vi "Read Dashboard Variables.vi"() -> ()   [LabVIEW 2020]
uses:
  <vilib>/Rock Robotics/Network Tables/NT Read Number.vi
  Framework/Robot Global Data.vi
panel:
  out "Transfer Release Duration":dbl
  out "Transfer Up Duration":dbl
  out "Intake Duration":dbl
  out "Shooter Duration":dbl
  out "Transfer Release Setpoint":dbl
  out "Transfer Up Setpoint":dbl
  out "Intake Setpoint":dbl
  out "Shooter Setpoint":dbl
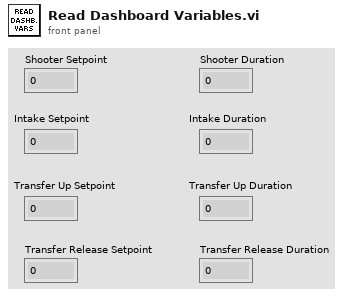
[diagram p1: front panel]
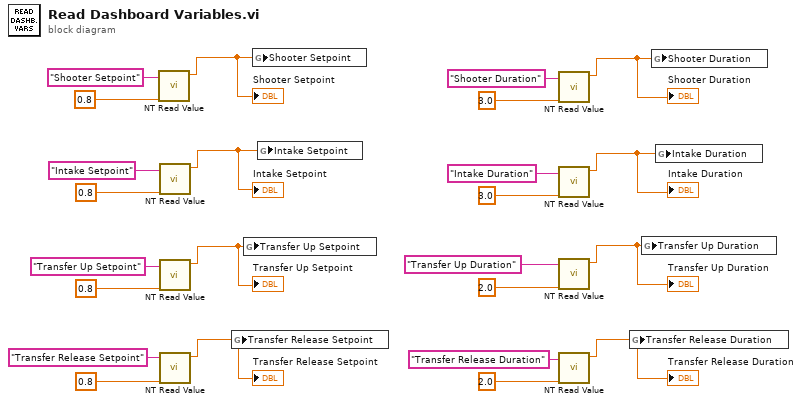
[diagram p0: block diagram]
diagram:
  n1 = call-poly <vilib>:"NT Read Value.vi"("Default Value"=0.8, "Name"="Shooter Setpoint") -> ("Numeric"=w22:dbl)  [unwired: 8 in, 1 out]
  "Shooter Setpoint" <- w22
  n2 = call-poly <vilib>:"NT Read Value.vi"("Default Value"=0.8, "Name"="Intake Setpoint") -> ("Numeric"=w7:dbl)  [unwired: 8 in, 1 out]
  "Intake Setpoint" <- w7
  n3 = call-poly <vilib>:"NT Read Value.vi"("Default Value"=0.8, "Name"="Transfer Up Setpoint") -> ("Numeric"=w6:dbl)  [unwired: 8 in, 1 out]
  "Transfer Up Setpoint" <- w6
  n4 = call-poly <vilib>:"NT Read Value.vi"("Default Value"=0.8, "Name"="Transfer Release Setpoint") -> ("Numeric"=w5:dbl)  [unwired: 8 in, 1 out]
  "Transfer Release Setpoint" <- w5
  n5 = global write "Robot Global Data.vi" "Transfer Release Setpoint"(w5) -> ()
  n6 = global write "Robot Global Data.vi" "Transfer Up Setpoint"(w6) -> ()
  n7 = global write "Robot Global Data.vi" "Shooter Setpoint"(w22) -> ()
  n8 = global write "Robot Global Data.vi" "Intake Setpoint"(w7) -> ()
  n9 = call-poly <vilib>:"NT Read Value.vi"("Default Value"=3.0, "Name"="Shooter Duration") -> ("Numeric"=w1:dbl)  [unwired: 8 in, 1 out]
  "Shooter Duration" <- w1
  n10 = call-poly <vilib>:"NT Read Value.vi"("Default Value"=3.0, "Name"="Intake Duration") -> ("Numeric"=w2:dbl)  [unwired: 8 in, 1 out]
  "Intake Duration" <- w2
  n11 = call-poly <vilib>:"NT Read Value.vi"("Default Value"=2.0, "Name"="Transfer Up Duration") -> ("Numeric"=w3:dbl)  [unwired: 8 in, 1 out]
  "Transfer Up Duration" <- w3
  n12 = call-poly <vilib>:"NT Read Value.vi"("Default Value"=2.0, "Name"="Transfer Release Duration") -> ("Numeric"=w4:dbl)  [unwired: 8 in, 1 out]
  "Transfer Release Duration" <- w4
  n13 = global write "Robot Global Data.vi" "Transfer Release Duration"(w4) -> ()
  n14 = global write "Robot Global Data.vi" "Transfer Up Duration"(w3) -> ()
  n15 = global write "Robot Global Data.vi" "Shooter Duration"(w1) -> ()
  n16 = global write "Robot Global Data.vi" "Intake Duration"(w2) -> ()
